vi "Proton's Energy.vi"(11 "Starting Velocity":dbl) -> (1 "Kinetic Energy":dbl, 3 "Energy":dbl)   [LabVIEW 2020]
doc: "[Prototype] This SubVi is purpose is to compute energy and kinetic energy of proton."
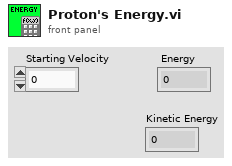
[diagram p1: front panel]
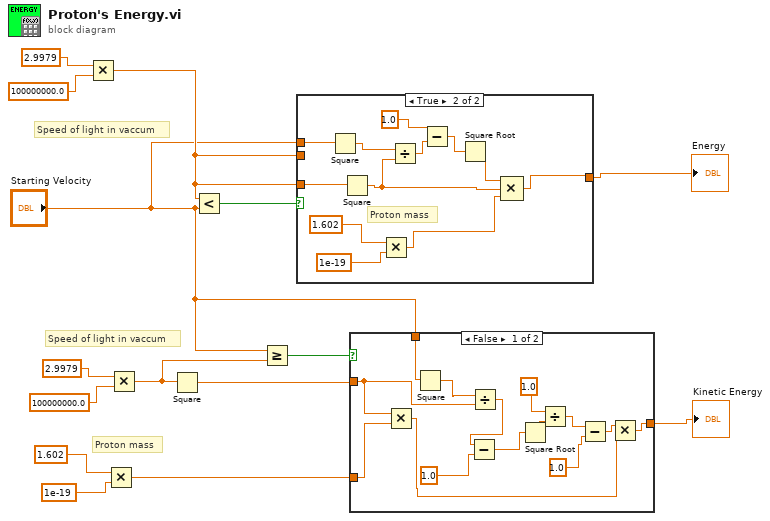
[diagram p0: block diagram]
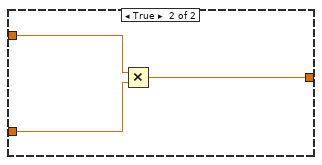
[diagram p2: hidden frame]
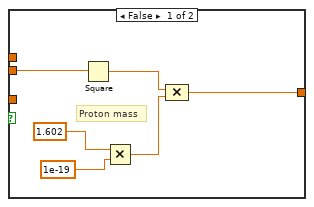
[diagram p3: hidden frame]
diagram:
  # "Speed of light in vaccum"
  # "Proton mass"
  # "Speed of light in vaccum"
  n1 = Multiply(x=2.9979, y=100000000.0) -> (x*y=w12:dbl)
  n2 = Multiply(x=1.602, y=1e-19) -> (x*y=w3:dbl)
  n3 = Multiply(x=2.9979, y=100000000.0) -> (x*y=w6:dbl)
  n4 = Square(x=w6) -> (x^2=w4:dbl)
  n5 = Less?(x=w12, y="Starting Velocity") -> (x < y?=w13:bool)
  n6 = Greater Or Equal?(x="Starting Velocity", y=w6) -> (x >= y?=w5:bool)
  n7 = case shown="True" w13 {
    tunnel: w12 -> [_ w30]
    tunnel: "Starting Velocity" -> [_ w23]
    tunnel: [w21 w22] -> w11
    tunnel: w12 -> [w16 _]
    frame False {
      # "Proton mass"
      n8 = Square(x=w16) -> (x^2=w17:dbl)
      n9 = Multiply(x=1.602, y=1e-19) -> (x*y=w18:dbl)
      n10 = Compound Arithmetic op=MULTIPLY(w17, w18) -> (w21:dbl)
    }
    frame True {
      # "Proton mass"
      n11 = Square(x=w23) -> (x^2=w24:dbl)
      n12 = Square(x=w30) -> (x^2=w25:dbl)
      n13 = Multiply(x=1.602, y=1e-19) -> (x*y=w31:dbl)
      n14 = Divide(x=w24, y=w25) -> (x/y=w27:dbl)
      n15 = Subtract(x=1.0, y=w27) -> (x-y=w26:dbl)
      n16 = Square Root(x=w26) -> (sqrt(x)=w29:dbl)
      n17 = Compound Arithmetic op=MULTIPLY(w29, w25, w31) -> (w22:dbl)
    }
  }
  "Energy" <- w11
  n18 = case shown="False" w5 {
    tunnel: w4 -> [w37 w50]
    tunnel: w3 -> [w47 w49]
    tunnel: [w36 w48] -> w2
    tunnel: "Starting Velocity" -> [w38 _]
    frame False {
      n19 = Multiply(x=w37, y=w47) -> (x*y=w34:dbl)
      n20 = Square(x=w38) -> (x^2=w41:dbl)
      n21 = Divide(x=w41, y=w37) -> (x/y=w40:dbl)
      n22 = Subtract(x=w40, y=1.0) -> (x-y=w39:dbl)
      n23 = Square Root(x=w39) -> (sqrt(x)=w45:dbl)
      n24 = Divide(x=1.0, y=w45) -> (x/y=w43:dbl)
      n25 = Subtract(x=w43, y=1.0) -> (x-y=w35:dbl)
      n26 = Multiply(x=w35, y=w34) -> (x*y=w36:dbl)
    }
    frame True {
      n27 = Multiply(x=w50, y=w49) -> (x*y=w48:dbl)
    }
  }
  "Kinetic Energy" <- w2
